vi "Initialize.vi"(8 "error in":errorcluster, 11 "Key in":refnum<class "Key.lvclass">) -> (0 "error out":errorcluster, 3 "Key out":refnum<class "Key.lvclass">)   [LabVIEW 2021, in "Library.lvlib" / "Key.lvclass"]
uses:
  Key.lvclass
  Key.lvclass/Key.ctl
  <vilib>/Utility/config.llb/NI_LVConfig.lvlib
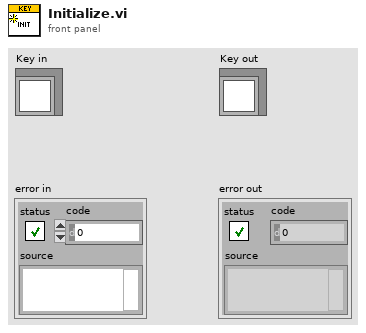
[diagram p1: front panel]
types:
  T1 = typedef "NI_LVConfig.lvlib/Config Data RefNum.ctl" = refnum<k1>
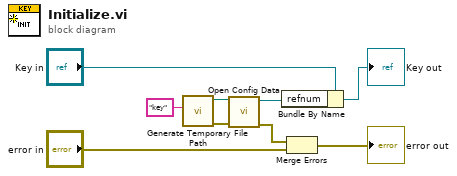
[diagram p0: block diagram]
diagram:
  n1 = call <vilib>:"Generate Temporary File Path.vi"("Temporary File Extension (tmp)"="key") -> ("error out"=w3:errorcluster, "Unique Temporary File Path"=w2:path)  [unwired: 9 in]
  n2 = call <vilib>:"Open Config Data.vi"("error in (no error)"=w3, "configuration file path"=w2) -> ("error out"=w4:errorcluster, "refnum"=w6:T1)  [unwired: 7 in, 1 out]
  n3 = Bundle By Name(cluster="Key in", "refnum"=w6) -> (→"Key out":refnum<class "Key.lvclass">)
  n4 = Merge Errors(w4, "error in") -> (→"error out":errorcluster)
